vi "ep_Synchronize Time.vi"(0 "RT controler time in":timestamp, 1 "reset":bool, 5 "maximum time difference (sec)":dbl=5.0 format="%#.6g", 7 "sampling rate (Hz)":dbl=9600.0 format="%#.6g", 9 "basic calc. interval (samples)":i32) -> (4 "RT controler time out":timestamp)   [LabVIEW 2011]
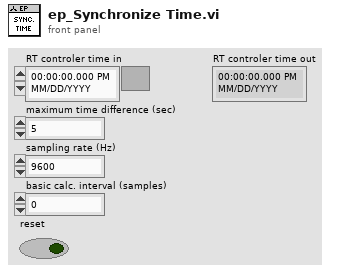
[diagram p1: front panel]
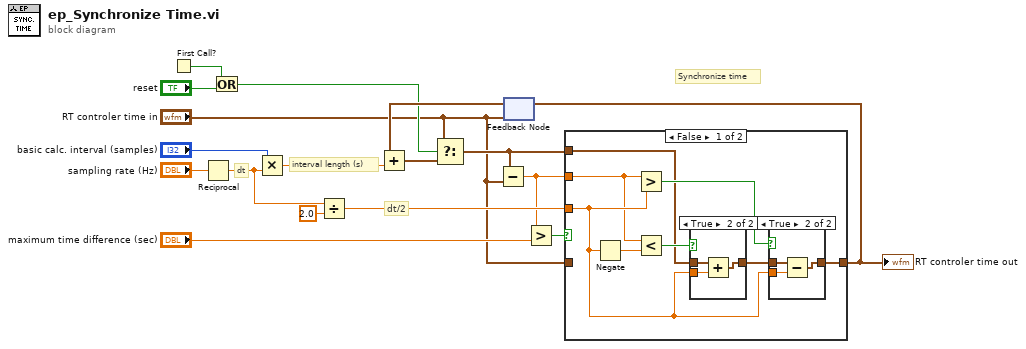
[diagram p0: block diagram]
diagram:
  # "Synchronize time"
  # "dt/2"
  # "dt"
  # "interval length (s)"
  n1 = First Call?() -> (First Call?: T/F=w7:bool)
  n2 = Reciprocal(x="sampling rate (Hz)") -> (1/x=w14:dbl)
  n3 = Or(x=w7, y="reset") -> (x .or. y?=w6:bool)
  n4 = Multiply(x="basic calc. interval (samples)", y=w14) -> (x*y=w16:dbl)
  n5 = Divide(x=w14, y=2.0) -> (x/y=w5:dbl)
  n6 = feedback #1("RT controler time in") -> (w17:timestamp)
  n7 = Add(x=w17, y=w16) -> (x+y=w15:timestamp)
  n8 = Select(t="RT controler time in", s=w6, f=w15) -> (s? t:f=w9:timestamp)
  n9 = Subtract(x=w9, y="RT controler time in") -> (x-y=w4:dbl)
  n10 = Greater?(x=w4, y="maximum time difference (sec)") -> (0:w2:bool)
  n11 = case shown="False" w2 {
    tunnel: [w25 w34] -> w12
    tunnel: w9 -> [w20 _]
    tunnel: w5 -> [w19 _]
    tunnel: w4 -> [w18 _]
    tunnel: "RT controler time in" -> [_ w34]
    frame False {
      n12 = Negate(x=w19) -> (-x=w24:dbl)
      n13 = Greater?(x=w18, y=w19) -> (0:w21:bool)
      n14 = Less?(x=w18, y=w24) -> (x < y?=w22:bool)
      n15 = case shown="True" w22 {
        tunnel: w20 -> [w26 w29]
        tunnel: w19 -> [_ w27]
        tunnel: [w26 w28] -> w23
        frame False {
        }
        frame True {
          n16 = Add(x=w29, y=w27) -> (x+y=w28:timestamp)
        }
      }
      n17 = case shown="True" w21 {
        tunnel: w23 -> [w30 w33]
        tunnel: w19 -> [_ w32]
        tunnel: [w30 w31] -> w25
        frame False {
        }
        frame True {
          n18 = Subtract(x=w33, y=w32) -> (x-y=w31:timestamp)
        }
      }
    }
    frame True {
    }
  }
  "RT controler time out" <- w12
  n19 = feedback-in #1(w12) -> ()
